vi "Replace or Add PJVS values into array of clusters.vi"(6 "index (0)":i32, 8 "PJVS reference voltages vector":dbl[](array[numeric]), 11 "PJVS reference voltages array of vector cluster":T1(array[cluster])) -> (3 "PJVS reference voltages array of vector cluster out":T1(array[cluster]))   [LabVIEW 2020]
doc: "Place PJVS array of voltages at proper place in Array of vector cluster.\nThis VI is because \"Replace Array Subset\" cannot replace array at position (index) outside of array dimension. I.e. it cannot enlarge array if needed."
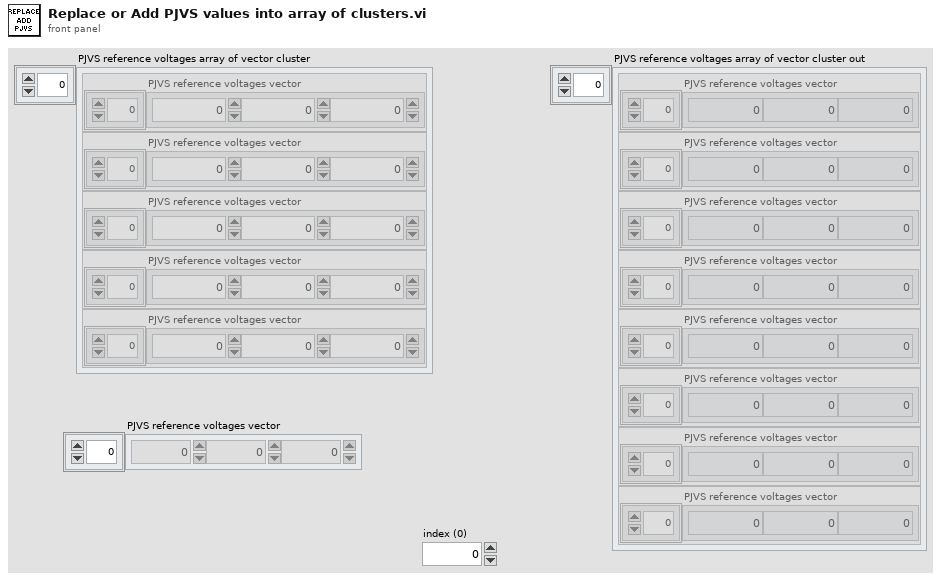
[diagram p1: front panel]
types:
  T1 = cluster{"PJVS reference voltages vector":dbl[]}[]
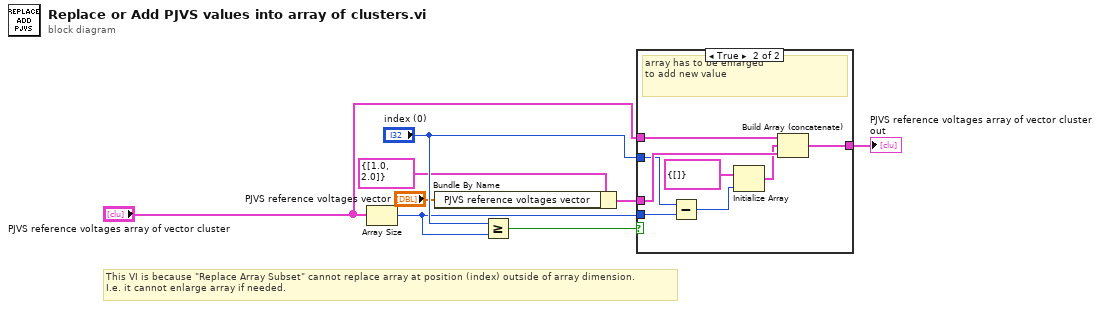
[diagram p0: block diagram]
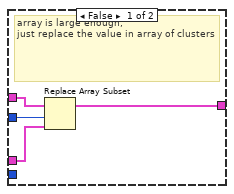
[diagram p2: hidden frame]
diagram:
  # "This VI is because \"Replace Array Subset\" cannot replace array at position (index) outside of array dimension.\nI.e. it cannot enlarge array if needed."
  n1 = Array Size(array="PJVS reference voltages array of vector cluster") -> (size(s)=w4:i32)
  n2 = Bundle By Name(cluster=cluster{"PJVS reference voltages vector":dbl[]} {"PJVS reference voltages vector"=[1.0, 2.0]} ("New PJVS reference voltages"), "PJVS reference voltages vector"="PJVS reference voltages vector") -> (w2:cluster{"PJVS reference voltages vector":dbl[]})
  n3 = Greater Or Equal?(x="index (0)", y=w4) -> (x >= y?=w5:bool)
  n4 = case shown="True" w5 {
    tunnel: "PJVS reference voltages array of vector cluster" -> [w12 w17]
    tunnel: "index (0)" -> [w11 w15]
    tunnel: w2 -> [w10 w19]
    tunnel: [w9 w16] -> w8
    tunnel: w4 -> [_ w14]
    frame False {
      # "array is large enough,\njust replace the value in array of clusters"
      n5 = Replace Array Subset(array=w12, new element=w10, index=w11) -> (w9:T1)
    }
    frame True {
      # "array has to be enlarged\nto add new value"
      n6 = Subtract(x=w15, y=w14) -> (x-y=w13:i32)
      n7 = Initialize Array(cluster{"PJVS reference voltages vector":dbl[]} {"PJVS reference voltages vector"=[]} ("new element/subarray"), w13) -> (w18:T1)
      n8 = Build Array (concatenate)(w17, w18, w19) -> (w16:T1)
    }
  }
  "PJVS reference voltages array of vector cluster out" <- w8
